vi "NTPModify2.vi"() -> ()   [LabVIEW 2023]
uses:
  <vilib>/Utility/file.llb/Write Delimited Spreadsheet (I64).vi
panel:
  in  "const + StdAvr":dbl
  out "AvrStd":dbl[](array[numeric])
  out "My std":dbl[](array[numeric]) format="%#_4g"
  out "Mean":dbl format="%.2f"
  out "Std":dbl format="%#_3g"
  out "Waveform Chart 4":dbl[][](graph) caption="Waveform Chart"
  out "Waveform Chart 3":dbl[][](graph) caption="Waveform Chart"
  out "Waveform Chart 2":u64[][](graph) caption="Waveform Chart"
  out "Waveform Chart":i64[][](graph)
  out "Numeric":i32
  out "last Date":string
  out "tmp64bit":i64[](array[numeric])
  in  "Statistic":bool
  out "StDeviation":dbl[](array[numeric]) format="%#_4g"
  in  "Matches Tab":enum32{"Page 1", "Page 2"}(tab)
  out "Table Control":string[][](table)
  out "appended array":string[](array[string])
  out "Mean by row":dbl[](array[numeric]) format="%.2f"
  out "Variance (xi - x) by row of 6@49":dbl[][](array[numeric])
  out "Last Draw":i64[](array[numeric])
  out "Matches":i32[][](array[numeric])
  out "Matches":i32[](array[numeric])
  out "Last Suppose":i32[][](array[numeric])
  out "Indicator":bool
  in  "Deviation":bool
  in  "Check":bool
  in  "Play":bool
  out "Your Suppose":i32[][](array[numeric])
  in  "Stop":bool
  # "V"
  # "G"
  # "Y"
  # "Last Suppose"
  # "Suppose Graph"
  # "Std Deviation"
  # "6@49"
  # "Your Suppose"
  # "Last Draw"
  # "Last Suppose"
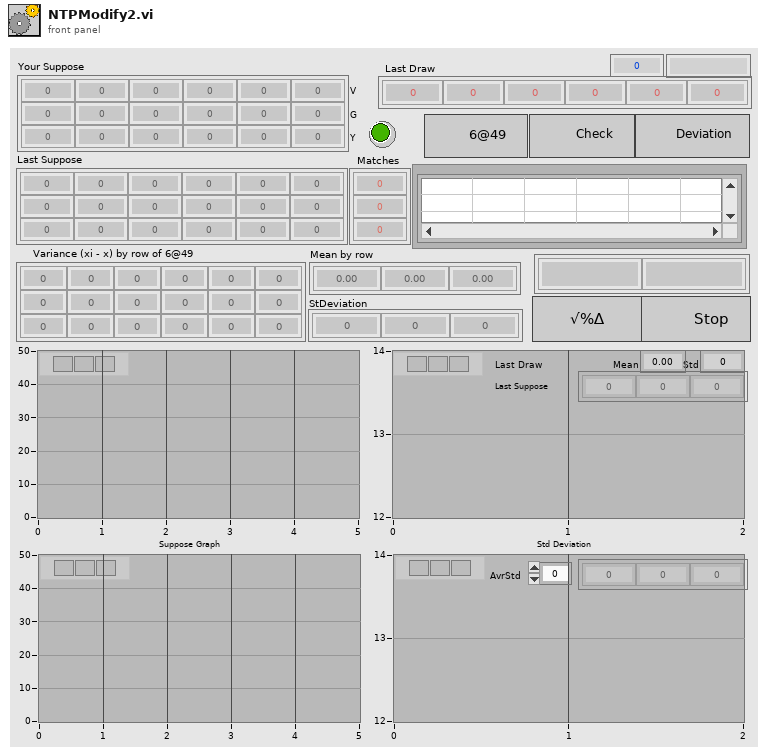
[diagram p1: front panel]
types:
  T1 = enum8{"Enabled", "Disabled", "Disabled and Grayed Out"}
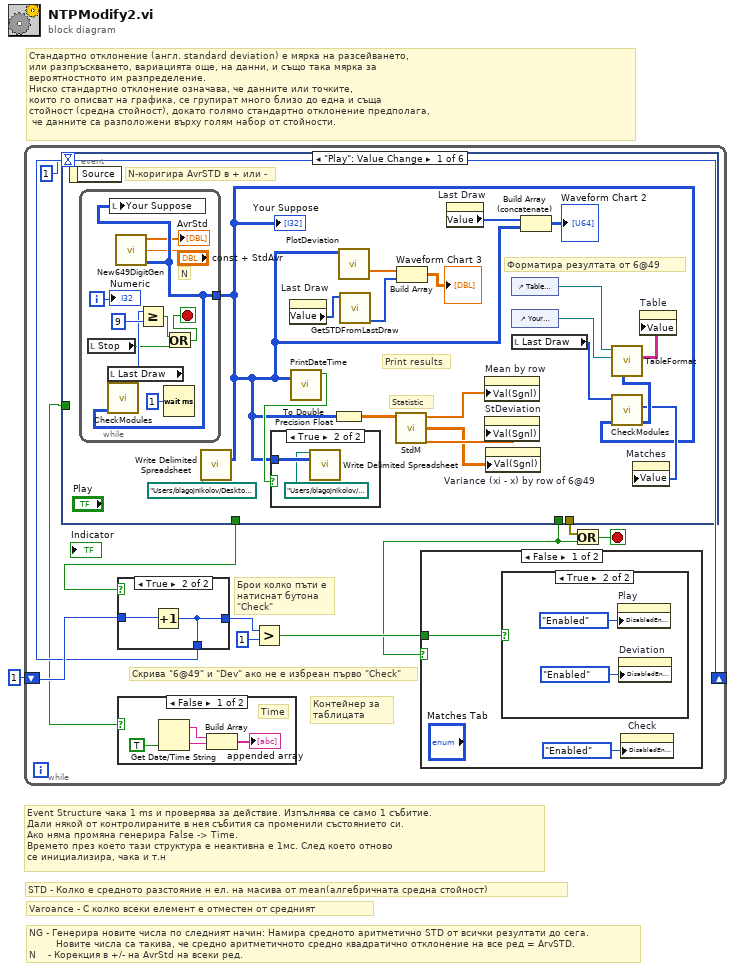
[diagram p0: block diagram]
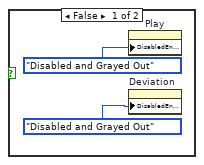
[diagram p4: hidden frame]
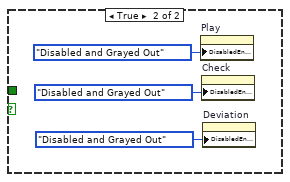
[diagram p5: hidden frame]
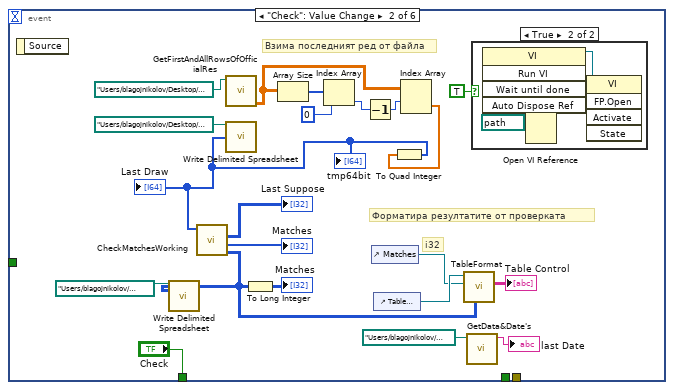
[diagram p7: hidden frame]
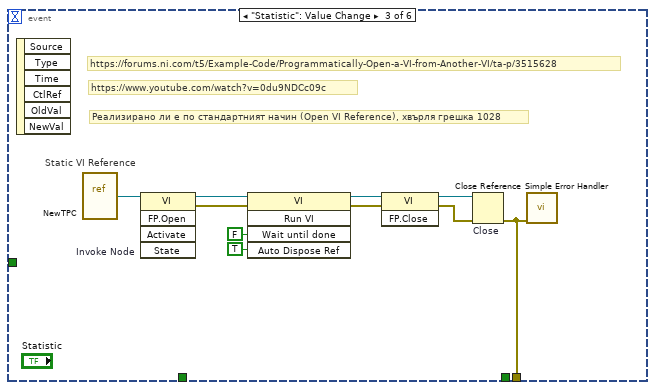
[diagram p9: hidden frame]
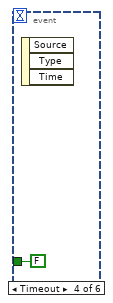
[diagram p10: hidden frame]
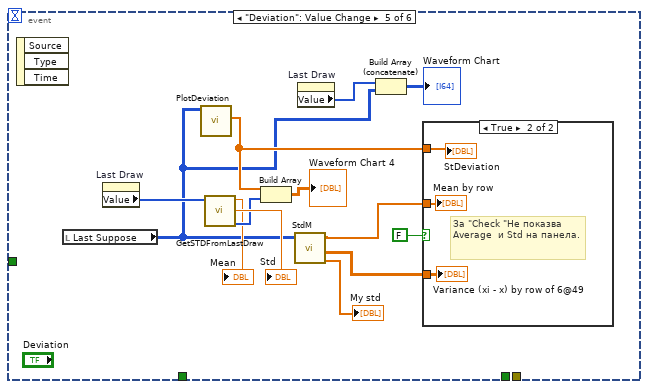
[diagram p11: hidden frame]
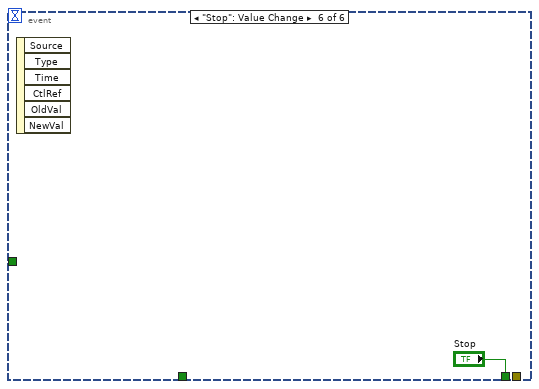
[diagram p13: hidden frame]
diagram:
  # "NG - Генерира новите числа по следният начин: Намира средното аритметично STD от всички резултати до сега.\n         Новите числа са такива, че средно аритметичното средно квадратично отклонение на все ред = ArvSTD. \nN    - Корекция в +/- на AvrStd на всеки ред."
  # "Varoance - С колко всеки елемент е отместен от средният"
  # "STD - Колко е средното разстояние н ел. на масива от mean(алгебричната средна стойност)"
  # "Event Structure чака 1 ms и проверява за действие. Изпълнява се само 1 събитие.\nДали някой от контролираните в нея събития са променили състоянието си.\nАко няма промяна генерира False -> Time.\nВремето през което тази структура е неактивна е 1мс. След което отново\nсе инициализира, чака и т.н"
  # "Стандартно отклонение (англ. standard deviation) е мярка на разсейването, \nили разпръскването, вариацията още, на данни, и също така мярка за \nвероятностното им разпределение. \nНиско стандартно отклонение означава, че данните или точките, \nкоито го описват на графика, се групират много близо до една и съща \nстойност (средна стойност), докато голямо стандартно отклонение предполага,\n че данните са разположени върху голям набор от стойности."
  n1 = while {
    shift-right: [w9] -> _
    shift-left: i64 1 -> [w11]
    stop <- w2 stop-if-true
    # "Скрива \"6@49\" и \"Dev\" ако не е избреан първо \"Check\""
    # "Брои колко пъти е\nнатиcнат бутона\n\"Check\""
    # "Контейнер за\nтаблицата"
    n2 = event shown="[0] \"Play\": Value Change" {
      selector: _ -> [_ _ _ _ _ _]
      dyn-events: _ -> [_ _ _ _ _ _]
      timeout: 1 -> [_ _ _ _ _ _]
      tunnel: [_ _ _ FALSE _ _] -> w6
      tunnel: [_ _ _ _ _ "Stop"] -> w4
      tunnel: [_ "Check" _ _ _ _] -> w5
      tunnel: [_ _ w87 _ _ _] -> w3
      event "Play": Value Change {
        # "N-коригира AvrSTD в + или -"
        # "Statistic"
        # "Форматира резултата от 6@49"
        # "Print results"
        n3 = event-data() -> ()  [unwired: 1 in, 1 out]
        n4 = while {
          tunnel: [w57] -> w29
          i -> [w55]
          stop <- w51 stop-if-true
          # "N"
          n5 = local read "Stop"() -> (w53:bool)
          n6 = local read "Last Draw"() -> (w58:i64[])
          n7 = call "New649DigitGen.vi"("const + StdAvr"="const + StdAvr") -> ("2D ResUArr - STD of each row is equal to (Last STD - Avr STD)"=w57:u64[][], "AvrSTDToArr - only six"=→"AvrStd":dbl[])  [unwired: 8 in, 1 out]
          n8 = call "CheckModules.vi"("Your Suppose"=w57, "Last Draw"=w58) -> ("sum"=w56:i32)  [unwired: 7 in, 2 out]
          n9 = local write "Your Suppose"(w57) -> ()
          n10 = Greater Or Equal?(x=w56, y=9) -> (x >= y?=w54:bool)
          n11 = Wait (ms)(milliseconds to wait=u32 1) -> ()  [unwired: 1 out]
          n12 = Or(x=w54, y=w53) -> (x .or. y?=w51:bool)
          "Numeric" <- w55
        }
        "Your Suppose" <- w29
        n13 = call-poly <vilib>:"Write Delimited Spreadsheet.vi"("file path (dialog if empty)"=path "/Users/blagojnikolov/Desktop/@tmp/tmp649Gen.txt", "2D data"=w29) -> ()  [unwired: 12 in, 2 out]
        n14 = property on="Last Draw" class="Arr (strict)"() -> ("Value"=w40:i64[])  [unwired: 2 in, 2 out]
        n15 = call "PrintDateTime.vi"("2D"=w29) -> ("T button?"=w46:bool)  [unwired: 10 in]
        n16 = case shown="True" w46 {
          tunnel: w29 -> [_ w49]
          frame False {
          }
          frame True {
            n17 = call-poly <vilib>:"Write Delimited Spreadsheet.vi"("file path (dialog if empty)"=path "/Users/blagojnikolov/Desktop/@tmp/archive.txt", "2D data"=w49) -> ()  [unwired: 12 in, 2 out]
          }
        }
        n18 = To Double Precision Float(number=w29) -> (double precision float=w30:dbl[][])
        n19 = call "PlotDeviation.vi"("Array"=w29) -> ("STD"=w43:dbl[])  [unwired: 7 in, 3 out]
        n20 = call "GetSTDFromLastDraw.vi"("Officials Results"=w40) -> ("StdRes array"=w42:u64[])  [unwired: 8 in, 2 out]
        n21 = call "StdM.vi"("2D"=w30) -> ("1D Std"=w32:dbl[], "[Xi-X]"=w31:dbl[][], "Mean"=w33:dbl[])  [unwired: 6 in, 2 out]
        n22 = Build Array(w43, w42) -> (→"Waveform Chart 3":dbl[][])
        n23 = property on="Last Draw" class="Arr (strict)"() -> ("Value"=w44:i64[])  [unwired: 2 in, 2 out]
        n24 = property on="Mean by row" class="Arr (strict)"("Val(Sgnl)"=w33) -> ()  [unwired: 2 in, 2 out]
        n25 = property on="StDeviation" class="Arr (strict)"("Val(Sgnl)"=w32) -> ()  [unwired: 2 in, 2 out]
        n26 = property on="Variance (xi - x) by row of 6@49" class="Arr (strict)"("Val(Sgnl)"=w31) -> ()  [unwired: 2 in, 2 out]
        n27 = control-ref of="Table Control"() -> (w39:refnum<vi>)
        n28 = control-ref of="Your Suppose"() -> (w35:refnum<vi>)
        n29 = local read "Last Draw"() -> (w34:i64[])
        n30 = Build Array (concatenate)(w44, w29) -> (→"Waveform Chart 2":u64[][])
        n31 = call "CheckModules.vi"("Your Suppose"=w29, "Last Draw"=w34) -> ("Matches"=w37:i32[][], "Matches 2"=w36:i32[])  [unwired: 7 in, 1 out]
        n32 = call "TableFormat.vi"("2D Double Array"=w37, "Arr Refnum"=w35, "Table in"=w39) -> ("TxtArray"=w38:string[][])  [unwired: 8 in]
        n33 = property on="Matches" class="Arr (strict)"("Value"=w36) -> ()  [unwired: 2 in, 2 out]
        n34 = property on="Table" class="Tbl (strict)"("Value"=w38) -> ()  [unwired: 2 in, 2 out]
      }
      event "Check": Value Change {
        # "Взима последният ред от файла"
        # "Форматира резултатите от проверката"
        # "i32"
        n35 = event-data() -> ()  [unwired: 1 in, 1 out]
        n36 = call "GetFirstAndAllRowsOfOfficialRes.vi"("file (use dialog)"=path "/Users/blagojnikolov/Desktop/@tmp/results.txt" ("file path (dialog if empty)")) -> ("All Officials Result"=w71:dbl[][])  [unwired: 8 in, 2 out]
        n37 = Array Size(array=w71) -> (size(s)=w69:i32[])
        n38 = Index Array(array=w69, index=0) -> (element=w70:i32)
        n39 = Decrement(x=w70) -> (x-1=w68:i32)
        n40 = control-ref of="Matches"() -> (w76:refnum<vi>)
        n41 = control-ref of="Table Control"() -> (w78:refnum<vi>)
        n42 = Index Array "Index Array"(array=w71, index (row)=w68) -> (element=w67:dbl[])  [unwired: 1 in]
        n43 = To Quad Integer(1:w67) -> (0:w66:i64[])
        "Last Draw" <- w66
        "tmp64bit" <- w66
        n44 = call "CheckMatchesWorking.vi"("Последен тираж"=w66) -> (0:w65:i64[][], "Съвпадения"=→"Matches":i32[], "Залози"=→"Last Suppose":i32[][])  [unwired: 7 in, 1 out]
        n45 = call-poly <vilib>:"Write Delimited Spreadsheet.vi"("file path (dialog if empty)"=path "/Users/blagojnikolov/Desktop/@tmp/matches.txt", "2D data"=w65) -> ()  [unwired: 12 in, 2 out]
        n46 = call-poly <vilib>:"Write Delimited Spreadsheet.vi"("file path (dialog if empty)"=path "/Users/blagojnikolov/Desktop/@tmp/officialResults.txt", "1D data"=w66) -> ()  [unwired: 12 in, 2 out]
        n47 = To Long Integer(number=w65) -> (32bit integer=→"Matches":i32[][])
        n48 = call "TableFormat.vi"("2D Double Array"=w65, "Arr Refnum"=w76, "Table in"=w78) -> ("TxtArray"=→"Table Control":string[][])  [unwired: 8 in]
        n49 = call "GetData&Date's.vi"("file: (fromSite.txt)"=path "/Users/blagojnikolov/Desktop/@tmp/fromSite.txt" ("file (use dialog)")) -> ("LastDate"=→"last Date":string)  [unwired: 8 in, 2 out]
        n50 = case shown="True" TRUE {
          frame False {
          }
          frame True {
            n51 = Open VI Reference(vi path=path "/Users/blagojnikolov/Library/Mobile Documents/com~apple~CloudDocs/» LabView/LabView/Project'24/Projects/649/AllAvrStdGraph.vi") -> (vi reference=w83:refnum<vi>)  [unwired: 5 in, 1 out]
            n52 = invoke on="Invoke Node" class="VI" method="Run VI"(reference=w83) -> (reference out=w82:refnum<vi>)  [unwired: 4 in, 4 out]
            n53 = invoke on="Invoke Node" class="VI" method="FP.Open"(reference=w82) -> ()  [unwired: 4 in, 5 out]
          }
        }
      }
      event "Statistic": Value Change {
        # "Static VI Reference"
        # "Реализирано ли е по стандартният начин (Open VI Reference), хвърля грешка 1028"
        # "https://www.youtube.com/watch?v=0du9NDCc09c"
        # "https://forums.ni.com/t5/Example-Code/Programmatically-Open-a-VI-from-Another-VI/ta-p/3515628"
        n54 = event-data() -> ()  [unwired: 1 in, 6 out]
        n55 = vi-ref "NewTPC.vi"() -> (w86:refnum<vi>)
        n56 = invoke on="Invoke Node" class="VI" method="FP.Open"(reference=w86) -> (reference out=w94:refnum<vi>, error out=w93:errorcluster)  [unwired: 4 in, 3 out]
        n57 = invoke class="VI" method="Run VI"(reference=w94, error in=w93, "Wait until done"=TRUE ("Wait Until Done"), "Auto Dispose Ref"=FALSE ("Auto Dispose Reference")) -> (reference out=w90:refnum<vi>, error out=w89:errorcluster)  [unwired: 1 in, 3 out]
        n58 = invoke class="VI" method="FP.Close"(reference=w90, error in=w89) -> (reference out=w85:refnum<vi>, error out=w88:errorcluster)  [unwired: 1 in, 1 out]
        n59 = Close Reference "Close"(reference=w85, error in (no error)=w88) -> (error out=w87:errorcluster)
        n60 = call <vilib>:"Simple Error Handler.vi"("error in (no error)"=w87) -> ()  [unwired: 4 in, 5 out]
      }
      event Timeout {
        n61 = event-data() -> ()  [unwired: 1 in, 3 out]
      }
      event "Deviation": Value Change {
        n62 = event-data() -> ()  [unwired: 1 in, 3 out]
        n63 = local read "Last Suppose"() -> (w99:i32[][])
        n64 = property on="Last Draw" class="Arr (strict)"() -> ("Value"=w106:i64[])  [unwired: 2 in, 2 out]
        n65 = call "PlotDeviation.vi"("Array"=w99) -> ("STD"=w102:dbl[])  [unwired: 7 in, 3 out]
        n66 = call "GetSTDFromLastDraw.vi"("Officials Results"=w106) -> ("StdRes array"=w103:u64[], "STD"=→"Std":dbl, "Mean"=→"Mean":dbl)  [unwired: 8 in]
        n67 = Build Array(w102, w103) -> (→"Waveform Chart 4":dbl[][])
        n68 = call "StdM.vi"("2D"=w99) -> ("1D Std"=→"My std":dbl[], "[Xi-X]"=w97:dbl[][], "Mean"=w98:dbl[])  [unwired: 6 in, 2 out]
        n69 = property on="Last Draw" class="Arr (strict)"() -> ("Value"=w107:i64[])  [unwired: 2 in, 2 out]
        n70 = Build Array (concatenate)(w107, w99) -> (→"Waveform Chart":i64[][])
        n71 = case shown="True" FALSE {
          tunnel: w97 -> [_ w111]
          tunnel: w102 -> [_ w110]
          tunnel: w98 -> [_ w109]
          frame False {
          }
          frame True {
            # "За \"Check \"Не показва Average  и Std на панела."
            "Variance (xi - x) by row of 6@49" <- w111
            "Mean by row" <- w109
            "StDeviation" <- w110
          }
        }
      }
      event "Stop": Value Change {
        n72 = event-data() -> ()  [unwired: 1 in, 6 out]
      }
    }
    n73 = case shown="True" w5 {
      tunnel: [w17 w18] -> w10
      tunnel: [w17 w18] -> w9
      tunnel: w11 -> [w17 w19]
      frame False {
      }
      frame True {
        n74 = Increment(x=w19) -> (x+1=w18:i64)
      }
    }
    n75 = case shown="False" w6 {
      frame False {
        # "Time"
        n76 = Get Date/Time String(want seconds? (F)=TRUE) -> (date string=w14:string, time string=w15:string)  [unwired: 2 in]
        n77 = Build Array(w14, w15) -> (→"appended array":string[])
      }
      frame True {
      }
    }
    n78 = Greater?(x=w10, y=i64 1) -> (0:w12:bool)
    n79 = case shown="False" w4 {
      tunnel: w12 -> [w20 _]
      frame False {
        n80 = case shown="True" w20 {
          frame False {
            n81 = property on="Play" class="Bool"("DisabledEnum"=T1."Disabled and Grayed Out" ("Disabled")) -> ()  [unwired: 2 in, 2 out]
            n82 = property on="Deviation" class="Bool"("DisabledEnum"=T1."Disabled and Grayed Out" ("Disabled")) -> ()  [unwired: 2 in, 2 out]
          }
          frame True {
            n83 = property on="Play" class="Bool"("DisabledEnum"=T1."Enabled" ("Disabled")) -> ()  [unwired: 2 in, 2 out]
            n84 = property on="Deviation" class="Bool"("DisabledEnum"=T1."Enabled" ("Disabled")) -> ()  [unwired: 2 in, 2 out]
          }
        }
        n85 = property on="Check" class="Bool"("DisabledEnum"=T1."Enabled" ("Disabled")) -> ()  [unwired: 2 in, 2 out]
      }
      frame True {
        n86 = property on="Play" class="Bool"("DisabledEnum"=T1."Disabled and Grayed Out" ("Disabled")) -> ()  [unwired: 2 in, 2 out]
        n87 = property on="Check" class="Bool"("DisabledEnum"=T1."Disabled and Grayed Out" ("Disabled")) -> ()  [unwired: 2 in, 2 out]
        n88 = property on="Deviation" class="Bool"("DisabledEnum"=T1."Disabled and Grayed Out" ("Disabled")) -> ()  [unwired: 2 in, 2 out]
      }
    }
    n89 = Or(x=w3, y=w4) -> (x .or. y?=w2:bool)
  }
